vi "Main.vi"(8 "error":errorcluster) -> (0 "Error out":errorcluster)   [LabVIEW 2018, in "S6.lvclass"]
doc: "Use this template to build a simple state machine design pattern. Each state executes code and determines which state to transition to."
uses:
  S6.lvclass
  S6.lvclass/S6.ctl
  Controller/Public Controls/GlobalConfig.ctl
  Controller/Public Controls/S2Config.ctl
  Public Controls/Outputs.ctl
  Controller/Public Controls/TestInfo.ctl
  Public Controls/ReportHeader.ctl
  62a9a080-f0ee-42f1-9851-61b6bd85b26e.vi
  18d9e863-2333-4af4-97b0-9e95cfa094dc.vi
  <vilib>/Utility/file.llb/Write Delimited Spreadsheet (string).vi
  Controller/GUI.lvclass
  IO/IO.lvclass
panel:
  out "Loop":i32
  # "S6 MAIN"
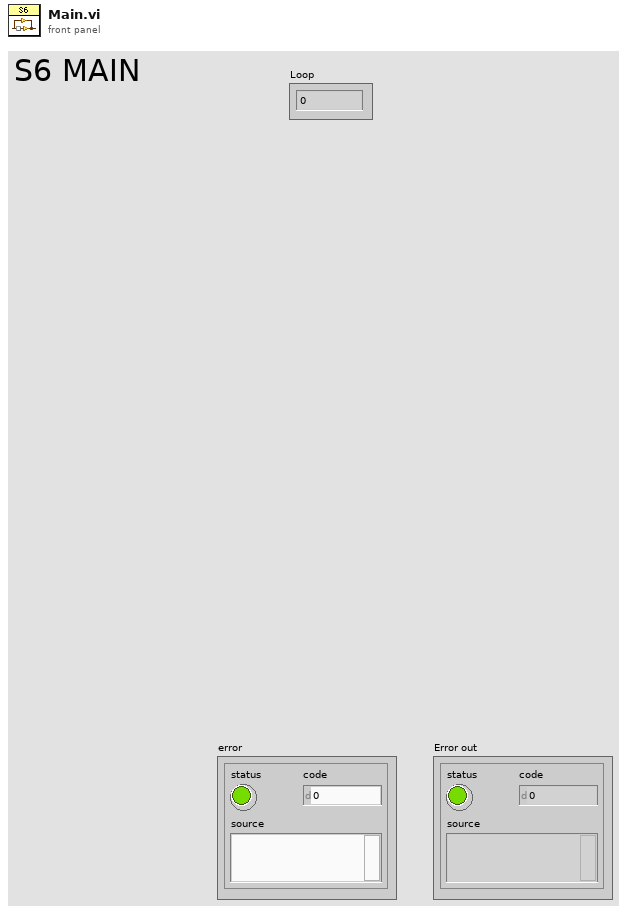
[diagram p1: front panel]
types:
  T1 = typedef "S6.lvclass/Outputs.ctl" = cluster{"LO P":bool, "HI P":bool, "Z3Vent":bool, "V2 Vent":bool, "IsLidLocked":bool}
  T2 = typedef "GUI.lvclass/TestInfo.ctl" = cluster{"TestType":string, "SN":string}
  T3 = typedef "S6.lvclass/ReportHeader.ctl" = string
  T4 = typedef "S6.lvclass/State.ctl" = enum16{"Initialize", "SetConfig", "AckAlarm", "Alarm", "Idle", "LockLid", "LowPressure", "Pressurize", "DecayTest", "Vent", "Abort", "Start", "CreateReports", "WriteToReport", "WritePressure", "Error", "Exit"}
  T5 = typedef "GUI.lvclass/S2Config.ctl" = cluster{"ECLOP_TIMER":dbl, "EC_PTEST_TIMER":dbl, "EC_PSTABLE_WAIT":dbl, "ECZ3_POFF_STABLE":dbl, "EC_PTEST_SCALE_FACTOR":dbl, "EC_PTEST_DELTA_BASELINE":dbl}
  T6 = typedef "GUI.lvclass/GlobalConfig.ctl" = cluster{"Report Folder Path":path, "PT1_MIN":dbl, "PT1_MAX":dbl, "VENT_PMAX":dbl, "LOP_TARGET":dbl, "LOP_RAMP":dbl, "LOP_LEAK_MAX":dbl, "HIP_TARGET":dbl, "HIP_RAMP":dbl, "HIP_MIN":dbl, "HIP_MAX":dbl, "BLEED_TIME":dbl, "LOP_MAX":dbl, "LOP_MIN":dbl, "PT131Com":refnum<visa-resource-name>, "PT231Com":refnum<visa-resource-name>, "PT331Com":refnum<visa-resource-name>, "PT431Com":refnum<visa-resource-name>, "PT531Com":refnum<visa-resource-name>, "PT631Com":refnum<visa-resource-name>}
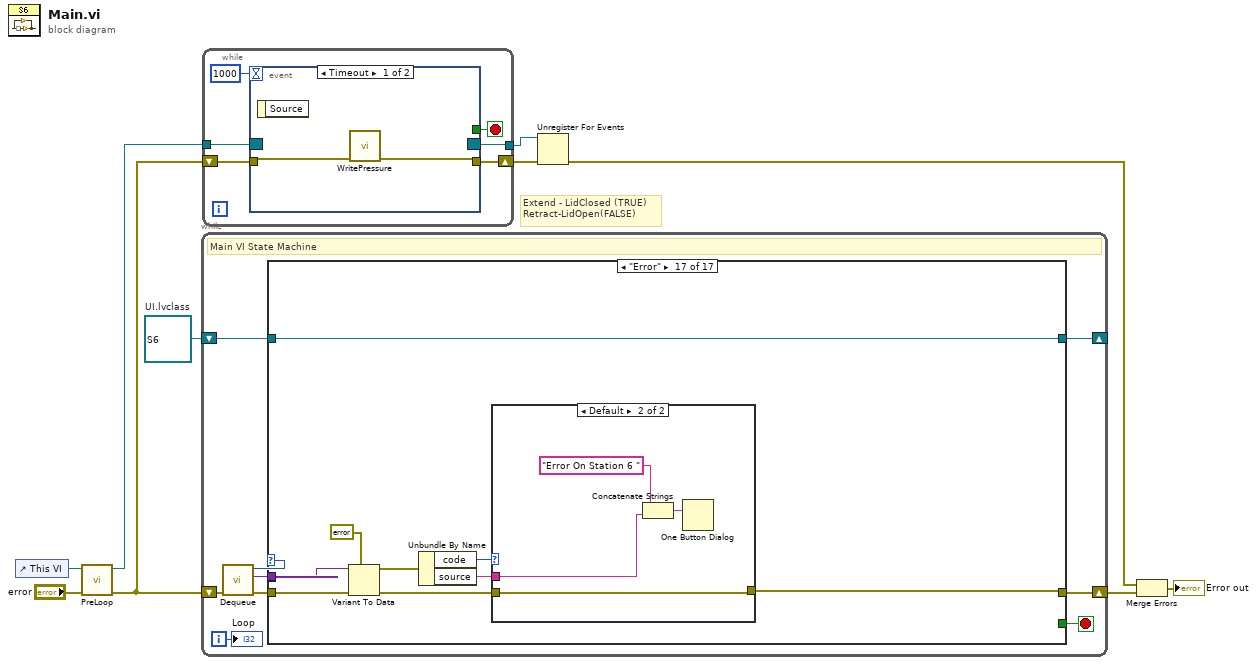
[diagram p0: block diagram]
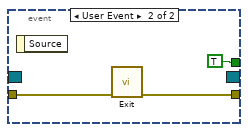
[diagram p2: hidden frame]
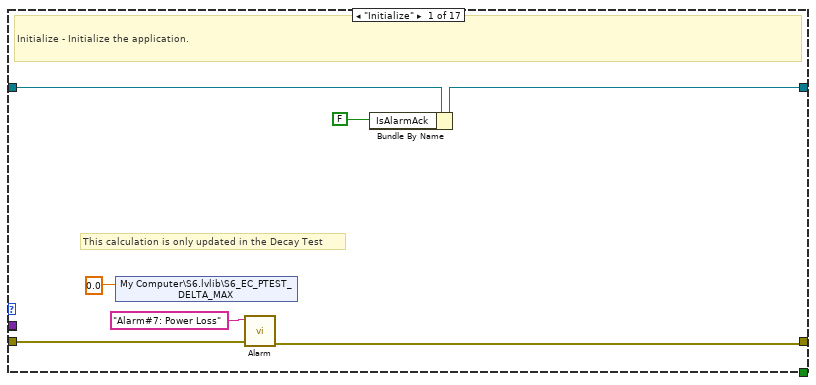
[diagram p3: hidden frame]
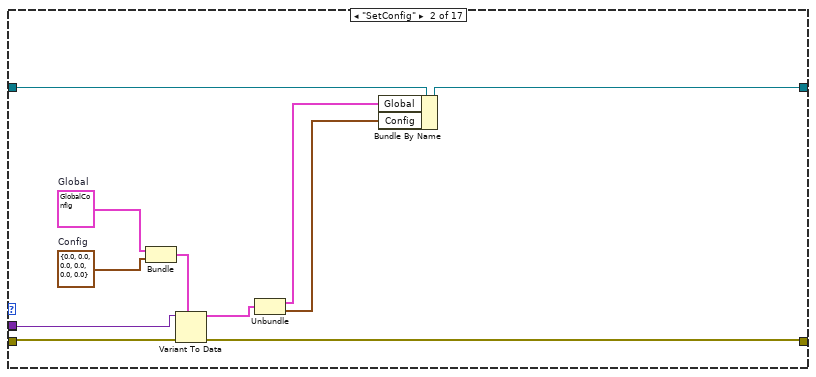
[diagram p4: hidden frame]
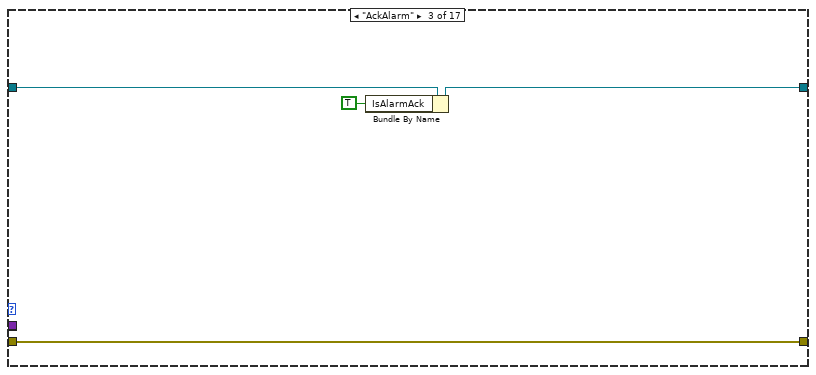
[diagram p5: hidden frame]
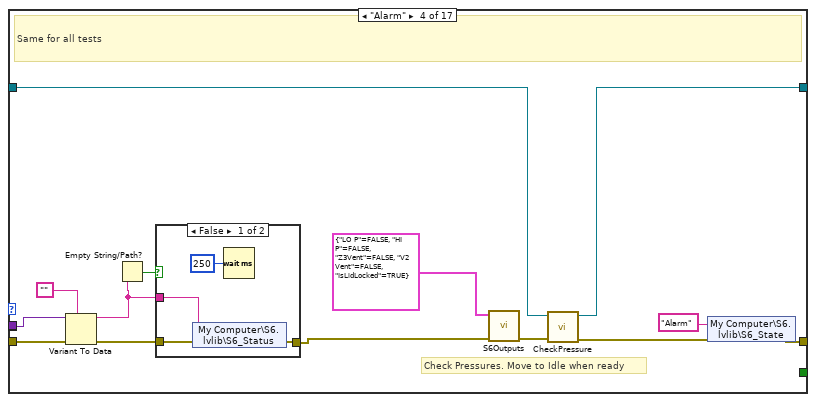
[diagram p6: hidden frame]
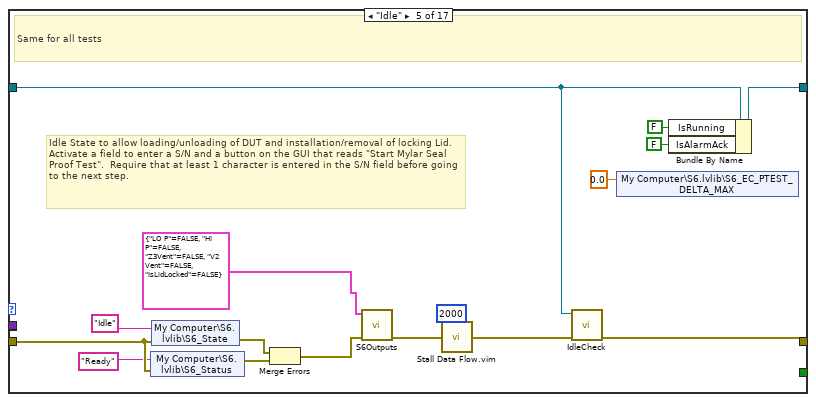
[diagram p8: hidden frame]
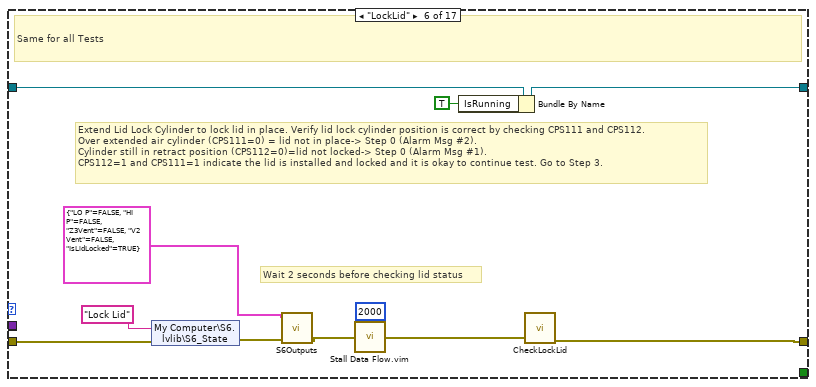
[diagram p9: hidden frame]
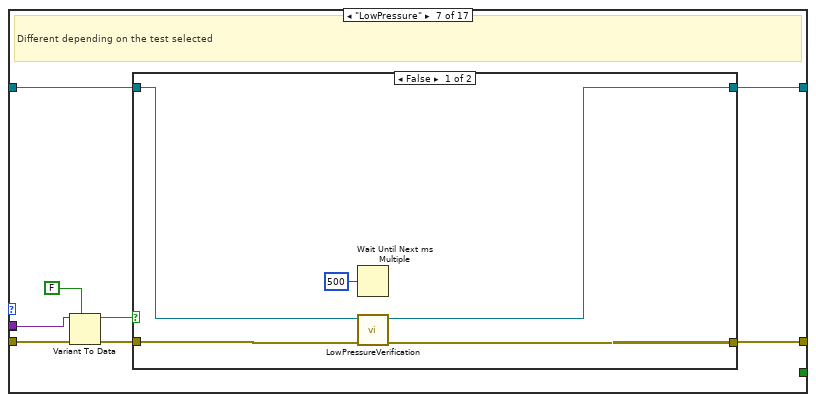
[diagram p10: hidden frame]
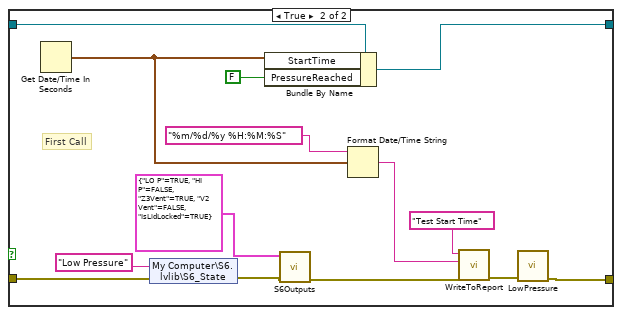
[diagram p11: hidden frame]
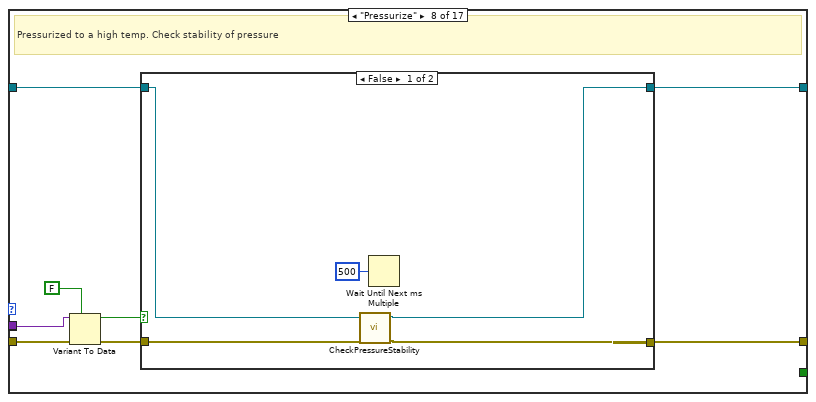
[diagram p12: hidden frame]
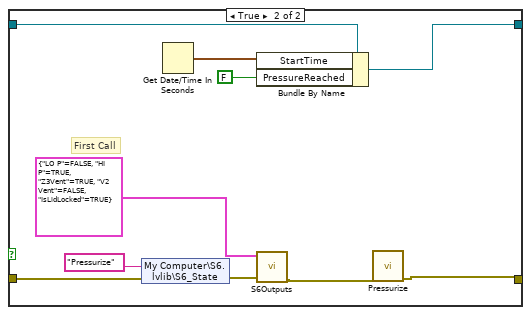
[diagram p13: hidden frame]
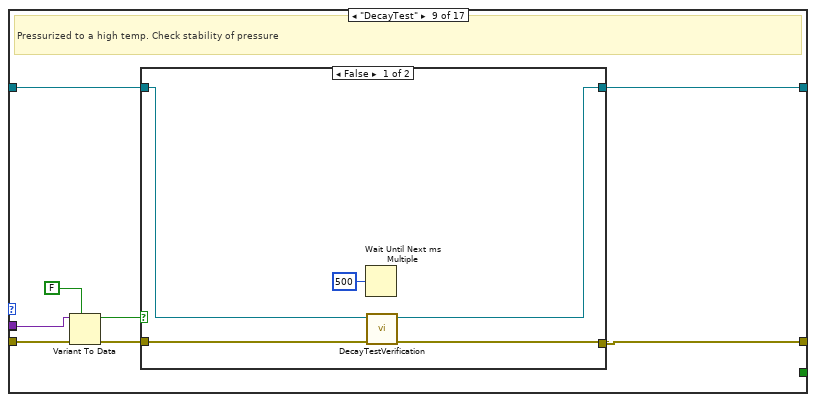
[diagram p14: hidden frame]
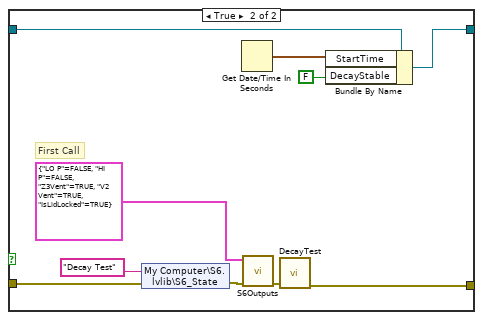
[diagram p15: hidden frame]
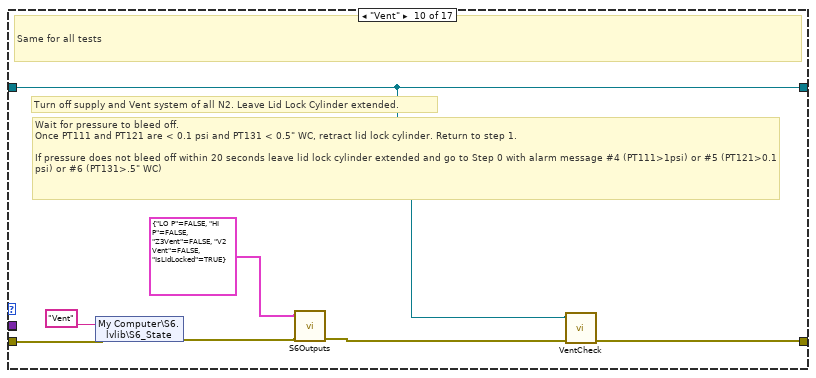
[diagram p16: hidden frame]
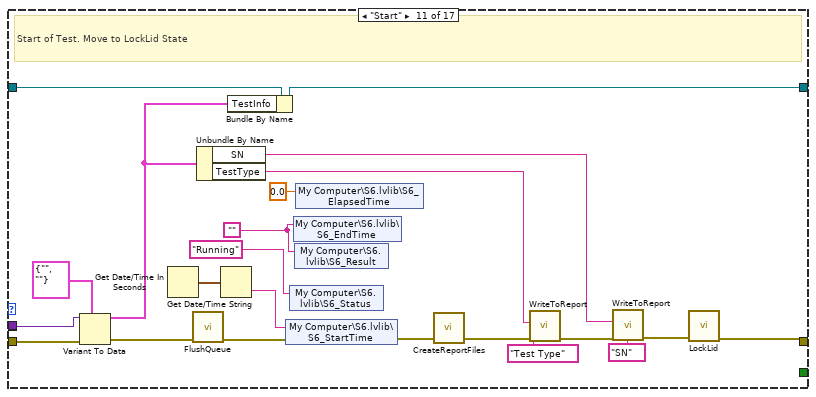
[diagram p17: hidden frame]
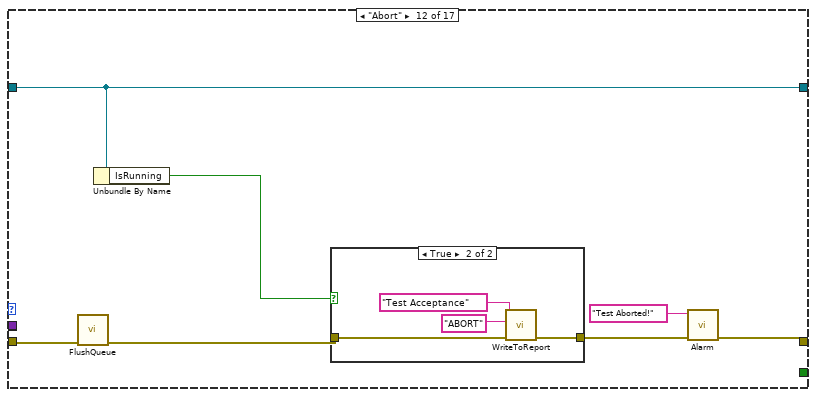
[diagram p18: hidden frame]
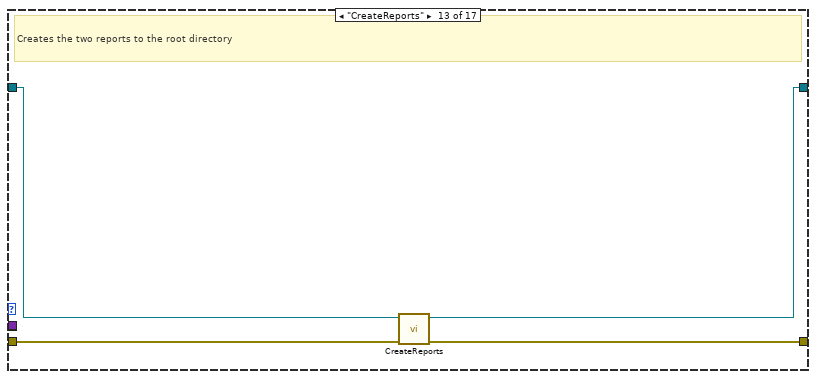
[diagram p20: hidden frame]
diagram:
  w10 = refnum<class "S6.lvclass"> refnum  # UI.lvclass
  # "Extend - LidClosed (TRUE)\nRetract-LidOpen(FALSE)"
  n1 = control-ref of="This VI"() -> (w7:refnum<vi>)
  n2 = call "PreLoop.vi"("error in"="error", "VI Ref"=w7) -> ("error out"=w6:errorcluster, "Event Registration Refnum"=w8:refnum<event-registration>)  [unwired: 8 in]
  n3 = while {
    shift-right: [w19] -> w3
    shift-left: w6 -> [w15]
    shift-right: [w16] -> _
    shift-left: w10 -> [w17]
    i -> [w11]
    stop <- w18 stop-if-true
    # "Main VI State Machine"
    n4 = call "Dequeue.vi"("error in"=w15) -> ("error out"=w14:errorcluster, "Data"=w12:variant, "State"=w13:T4)  [unwired: 8 in]
    n5 = case shown="\"Error\"" w13 {
      tunnel: [_ _ _ _ _ _ _ _ _ _ _ _ _ _ _ w244 _] -> w18
      tunnel: w14 -> [w24 w36 w41 w50 w75 w86 w94 w121 w144 w167 w185 w190 w204 w218 w223 w242 w250]
      tunnel: [w23 w27 w41 w51 w69 w84 w95 w122 w145 w165 w174 w195 w203 w211 w222 w242 w246] -> w19
      tunnel: w17 -> [w26 w37 w40 w54 w65 w87 w89 w116 w139 w164 w189 w194 w205 w217 w225 w243 w253]
      tunnel: [w25 w31 w39 w53 w71 w81 w88 w115 w138 w164 w182 w194 w202 w217 w225 w243 w253] -> w16
      tunnel: w12 -> [_ w32 _ w49 _ _ w93 w120 w143 _ w183 _ _ w219 _ _ w249]
      tunnel: w12 -> [_ _ _ _ _ _ _ _ _ _ _ _ _ _ _ _ _]
      frame "Initialize" {
        # "This calculation is only updated in the Decay Test"
        # "Initialize - Initialize the application."
        n6 = shared-variable "My Computer\\S6.lvlib\\S6_EC_PTEST_DELTA_MAX"(0.0 ("EC_PTEST_DELTA_MAX")) -> ()  [unwired: 1 in, 1 out]
        n7 = call "Alarm.vi"("error in"=w24, "Alarm"="Alarm#7: Power Loss" ("Status")) -> ("error out"=w23:errorcluster)  [unwired: 9 in]
        n8 = Bundle By Name(cluster=w26, "IsAlarmAck"=FALSE) -> (w25:refnum<class "S6.lvclass">)
      }
      frame "SetConfig" {
        w34 = T5 {"ECLOP_TIMER"=0.0, "EC_PTEST_TIMER"=0.0, "EC_PSTABLE_WAIT"=0.0, "ECZ3_POFF_STABLE"=0.0, "EC_PTEST_SCALE_FACTOR"=0.0, "EC_PTEST_DELTA_BASELINE"=0.0}  # Config
        w35 = T6 {"Report Folder Path"=path "", "PT1_MIN"=0.0, "PT1_MAX"=0.0, "VENT_PMAX"=0.0, "LOP_TARGET"=0.0, "LOP_RAMP"=0.0, "LOP_LEAK_MAX"=0.0, "HIP_TARGET"=0.0, "HIP_RAMP"=0.0, "HIP_MIN"=0.0, "HIP_MAX"=0.0, "BLEED_TIME"=0.0, "LOP_MAX"=0.0, "LOP_MIN"=0.0, "PT131Com"="COM5", "PT231Com"="COM6", "PT331Com"="COM7", "PT431Com"="COM8", "PT531Com"="COM9", "PT631Com"="COM10"}  # Global
        n9 = Bundle("Global"=w35, "Config"=w34) -> (w33:cluster{"Global":T6, "Config":T5})  [unwired: 1 in]
        n10 = Variant To Data(error in=w36, type=w33, Variant=w32) -> (data=w30:cluster{"Global":T6, "Config":T5}, error out=w27:errorcluster)
        n11 = Unbundle(w30) -> ("Global"=w29:T6, "Config"=w28:T5)
        n12 = Bundle By Name(cluster=w37, "Global"=w29, "Config"=w28) -> (w31:refnum<class "S6.lvclass">)
      }
      frame "AckAlarm" {
        n13 = Bundle By Name(cluster=w40, "IsAlarmAck"=TRUE) -> (w39:refnum<class "S6.lvclass">)
      }
      frame "Alarm" {
        # "Check Pressures. Move to Idle when ready"
        # "Same for all tests"
        n14 = Variant To Data(error in=w50, type="", Variant=w49) -> (data=w46:string, error out=w45:errorcluster)
        n15 = Empty String/Path?(string/path=w46) -> (empty?=w47:bool)
        n16 = case shown="False" w47 {
          tunnel: w46 -> [w59 _]
          tunnel: w45 -> [w58 w60]
          tunnel: [w57 w60] -> w43
          frame False {
            n17 = shared-variable "My Computer\\S6.lvlib\\S6_Status"(w59, error in=w58) -> (error out=w57:errorcluster)
            n18 = Wait (ms)(milliseconds to wait=u32 250) -> ()  [unwired: 1 out]
          }
          frame True {
          }
        }
        n19 = call "S6Outputs.vi"("error in"=w43, "Outputs"=T1 {"LO P"=FALSE, "HI P"=FALSE, "Z3Vent"=FALSE, "V2 Vent"=FALSE, "IsLidLocked"=TRUE} ("SIOutputs")) -> ("error out"=w42:errorcluster)  [unwired: 9 in]
        n20 = call "CheckPressure.vi"("error in (no error)"=w42, "UI.lvclass"=w54) -> ("error out"=w52:errorcluster, "UI.lvclass 2"=w53:refnum<class "S6.lvclass">)  [unwired: 8 in]
        n21 = shared-variable "My Computer\\S6.lvlib\\S6_State"("Alarm" ("S1Status"), error in=w52) -> (error out=w51:errorcluster)
      }
      frame "Idle" {
        # "Idle State to allow loading/unloading of DUT and installation/removal of locking Lid.  Activate a field to enter a S/N and a button on the GUI that reads \"Start Mylar Seal Proof Test\".  Require that at least 1 character is entered in the S/N field before going to the next step."
        # "Same for all tests"
        n22 = shared-variable "My Computer\\S6.lvlib\\S6_Status"("Ready" ("Status"), error in=w75) -> (error out=w73:errorcluster)
        n23 = shared-variable "My Computer\\S6.lvlib\\S6_State"("Idle" ("S1Status"), error in=w75) -> (error out=w74:errorcluster)
        n24 = Merge Errors(w74, w73) -> (w62:errorcluster)
        n25 = call "S6Outputs.vi"("error in"=w62, "Outputs"=T1 {"LO P"=FALSE, "HI P"=FALSE, "Z3Vent"=FALSE, "V2 Vent"=FALSE, "IsLidLocked"=FALSE} ("SIOutputs")) -> ("error out"=w61:errorcluster)  [unwired: 9 in]
        n26 = call "Stall Data Flow.vim"("value in"=w61, "milliseconds to wait"=u32 2000) -> ("value out"=w67:errorcluster)  [unwired: 1 out]
        n27 = call "IdleCheck.vi"("error in (no error)"=w67, "S2.lvclass"=w65) -> ("error out"=w69:errorcluster)  [unwired: 9 in]
        n28 = shared-variable "My Computer\\S6.lvlib\\S6_EC_PTEST_DELTA_MAX"(0.0 ("EC_PTEST_DELTA_MAX")) -> ()  [unwired: 1 in, 1 out]
        n29 = Bundle By Name(cluster=w65, "IsRunning"=FALSE, "IsAlarmAck"=FALSE) -> (w71:refnum<class "S6.lvclass">)
      }
      frame "LockLid" {
        # "Wait 2 seconds before checking lid status"
        # "Extend Lid Lock Cylinder to lock lid in place. Verify lid lock cylinder position is correct by checking CPS111 and CPS112. \nOver extended air cylinder (CPS111=0) = lid not in place-> Step 0 (Alarm Msg #2). \nCylinder still in retract position (CPS112=0)=lid not locked-> Step 0 (Alarm Msg #1). \nCPS112=1 and CPS111=1 indicate the lid is installed and locked and it is okay to continue test. Go to Step 3."
        # "Same for all Tests"
        n30 = shared-variable "My Computer\\S6.lvlib\\S6_State"("Lock Lid" ("S1Status"), error in=w86) -> (error out=w78:errorcluster)
        n31 = call "S6Outputs.vi"("error in"=w78, "Outputs"=T1 {"LO P"=FALSE, "HI P"=FALSE, "Z3Vent"=FALSE, "V2 Vent"=FALSE, "IsLidLocked"=TRUE} ("SIOutputs")) -> ("error out"=w77:errorcluster)  [unwired: 9 in]
        n32 = call "Stall Data Flow.vim"("value in"=w77, "milliseconds to wait"=u32 2000) -> ("value out"=w83:errorcluster)  [unwired: 1 out]
        n33 = Bundle By Name(cluster=w87, "IsRunning"=TRUE) -> (w81:refnum<class "S6.lvclass">)
        n34 = call "CheckLockLid.vi"("error in (no error)"=w83) -> ("error out"=w84:errorcluster)  [unwired: 10 in]
      }
      frame "LowPressure" {
        # "Different depending on the test selected"
        n35 = Variant To Data(error in=w94, type=FALSE, Variant=w93) -> (data=w90:bool, error out=w91:errorcluster)
        n36 = case shown="False" w90 {
          tunnel: [w99 w104] -> w95
          tunnel: w91 -> [w100 w113]
          tunnel: w89 -> [w98 w110]
          tunnel: [w97 w112] -> w88
          frame False {
            n37 = Wait Until Next ms Multiple(millisecond multiple=u32 500) -> ()  [unwired: 1 out]
            n38 = call "LowPressureVerification.vi"("error in"=w100, "S1 in"=w98) -> ("error out"=w99:errorcluster, "S1 out"=w97:refnum<class "S6.lvclass">)  [unwired: 8 in]
          }
          frame True {
            # "First Call"
            n39 = Get Date/Time In Seconds() -> (seconds since 1Jan1904=w107:timestamp)
            n40 = shared-variable "My Computer\\S6.lvlib\\S6_State"("Low Pressure" ("S1Status"), error in=w113) -> (error out=w102:errorcluster)
            n41 = Bundle By Name(cluster=w110, "StartTime"=w107, "PressureReached"=FALSE ("PT111ReachedPressure")) -> (w112:refnum<class "S6.lvclass">)
            n42 = call "S6Outputs.vi"("error in"=w102, "Outputs"=T1 {"LO P"=TRUE, "HI P"=FALSE, "Z3Vent"=TRUE, "V2 Vent"=FALSE, "IsLidLocked"=TRUE} ("SIOutputs")) -> ("error out"=w101:errorcluster)  [unwired: 9 in]
            n43 = Format Date/Time String(time format string (%c)="%m/%d/%y %H:%M:%S", seconds (now)=w107) -> (date/time string=w106:string)  [unwired: 1 in]
            n44 = call "WriteToReport.vi"("error in"=w101, "Value"=w106, "Header"="Test Start Time" ("S1Status")) -> ("error out"=w105:errorcluster)  [unwired: 8 in]
            n45 = call "LowPressure.vi"("error in"=w105) -> ("error out"=w104:errorcluster)  [unwired: 10 in]
          }
        }
      }
      frame "Pressurize" {
        # "Pressurized to a high temp. Check stability of pressure"
        n46 = Variant To Data(error in=w121, type=FALSE, Variant=w120) -> (data=w117:bool, error out=w118:errorcluster)
        n47 = case shown="False" w117 {
          tunnel: [w124 w131] -> w122
          tunnel: w118 -> [w125 w136]
          tunnel: w116 -> [w127 w132]
          tunnel: [w126 w135] -> w115
          frame False {
            n48 = call "CheckPressureStability.vi"("error in"=w125, "S1 in"=w127) -> ("error out"=w124:errorcluster, "S1 out"=w126:refnum<class "S6.lvclass">)  [unwired: 8 in]
            n49 = Wait Until Next ms Multiple(millisecond multiple=u32 500) -> ()  [unwired: 1 out]
          }
          frame True {
            # "First Call"
            n50 = shared-variable "My Computer\\S6.lvlib\\S6_State"("Pressurize" ("S1Status"), error in=w136) -> (error out=w129:errorcluster)
            n51 = Get Date/Time In Seconds() -> (seconds since 1Jan1904=w134:timestamp)
            n52 = Bundle By Name(cluster=w132, "StartTime"=w134, "PressureReached"=FALSE ("PT111ReachedPressure")) -> (w135:refnum<class "S6.lvclass">)
            n53 = call "S6Outputs.vi"("error in"=w129, "Outputs"=T1 {"LO P"=FALSE, "HI P"=TRUE, "Z3Vent"=TRUE, "V2 Vent"=FALSE, "IsLidLocked"=TRUE} ("SIOutputs")) -> ("error out"=w128:errorcluster)  [unwired: 9 in]
            n54 = call "Pressurize.vi"("error in"=w128) -> ("error out"=w131:errorcluster)  [unwired: 10 in]
          }
        }
      }
      frame "DecayTest" {
        # "Pressurized to a high temp. Check stability of pressure"
        n55 = Variant To Data(error in=w144, type=FALSE, Variant=w143) -> (data=w140:bool, error out=w141:errorcluster)
        n56 = case shown="False" w140 {
          tunnel: [w147 w155] -> w145
          tunnel: w141 -> [w148 w159]
          tunnel: w139 -> [w150 w156]
          tunnel: [w149 w158] -> w138
          frame False {
            n57 = Wait Until Next ms Multiple(millisecond multiple=u32 500) -> ()  [unwired: 1 out]
            n58 = call "DecayTestVerification.vi"("error in"=w148, "ClassDataIn"=w150) -> ("error out"=w147:errorcluster, "S1 out"=w149:refnum<class "S6.lvclass">)  [unwired: 8 in]
          }
          frame True {
            # "First Call"
            n59 = shared-variable "My Computer\\S6.lvlib\\S6_State"("Decay Test" ("S1Status"), error in=w159) -> (error out=w152:errorcluster)
            n60 = Get Date/Time In Seconds() -> (seconds since 1Jan1904=w157:timestamp)
            n61 = call "S6Outputs.vi"("error in"=w152, "Outputs"=T1 {"LO P"=FALSE, "HI P"=FALSE, "Z3Vent"=TRUE, "V2 Vent"=TRUE, "IsLidLocked"=TRUE} ("SIOutputs")) -> ("error out"=w151:errorcluster)  [unwired: 9 in]
            n62 = call "DecayTest.vi"("error in"=w151) -> ("error out"=w155:errorcluster)  [unwired: 10 in]
            n63 = Bundle By Name(cluster=w156, "StartTime"=w157, "DecayStable"=FALSE) -> (w158:refnum<class "S6.lvclass">)
          }
        }
      }
      frame "Vent" {
        # "Wait for pressure to bleed off. \nOnce PT111 and PT121 are < 0.1 psi and PT131 < 0.5\" WC, retract lid lock cylinder. Return to step 1. \n\nIf pressure does not bleed off within 20 seconds leave lid lock cylinder extended and go to Step 0 with alarm message #4 (PT111>1psi) or #5 (PT121>0.1 psi) or #6 (PT131>.5\" WC)"
        # "Turn off supply and Vent system of all N2. Leave Lid Lock Cylinder extended."
        # "Same for all tests"
        n64 = shared-variable "My Computer\\S6.lvlib\\S6_State"("Vent" ("S1Status"), error in=w167) -> (error out=w162:errorcluster)
        n65 = call "S6Outputs.vi"("error in"=w162, "Outputs"=T1 {"LO P"=FALSE, "HI P"=FALSE, "Z3Vent"=FALSE, "V2 Vent"=FALSE, "IsLidLocked"=TRUE} ("SIOutputs")) -> ("error out"=w161:errorcluster)  [unwired: 9 in]
        n66 = call "VentCheck.vi"("error in (no error)"=w161, "S2.lvclass"=w164) -> ("error out"=w165:errorcluster)  [unwired: 9 in]
      }
      frame "Start" {
        w171 = ""
        # "Start of Test. Move to LockLid State"
        n67 = Variant To Data(error in=w185, type=T2 {"TestType"="", "SN"=""} ("TestInfo"), Variant=w183) -> (data=w179:T2, error out=w169:errorcluster)
        n68 = Get Date/Time In Seconds() -> (seconds since 1Jan1904=w188:timestamp)
        n69 = call "FlushQueue.vi"("error in"=w169) -> ("error out"=w168:errorcluster)  [unwired: 10 in]
        n70 = Unbundle By Name(w179) -> ("SN"=w177:string, "TestType"=w170:string)
        n71 = Get Date/Time String(seconds (now)=w188) -> (time string=w187:string)  [unwired: 2 in, 1 out]
        n72 = Bundle By Name(cluster=w189, "TestInfo"=w179) -> (w182:refnum<class "S6.lvclass">)
        n73 = shared-variable "My Computer\\S6.lvlib\\S6_StartTime"(w187, error in=w168) -> (error out=w173:errorcluster)
        n74 = shared-variable "My Computer\\S6.lvlib\\S6_Status"("Running" ("S1Status")) -> ()  [unwired: 1 in, 1 out]
        n75 = shared-variable "My Computer\\S6.lvlib\\S6_EndTime"(w171) -> ()  [unwired: 1 in, 1 out]
        n76 = shared-variable "My Computer\\S6.lvlib\\S6_Result"(w171) -> ()  [unwired: 1 in, 1 out]
        n77 = shared-variable "My Computer\\S6.lvlib\\S6_ElapsedTime"(0.0 ("ElapsedTime")) -> ()  [unwired: 1 in, 1 out]
        n78 = call "CreateReportFiles.vi"("error in"=w173) -> ("error out"=w180:errorcluster)  [unwired: 10 in]
        n79 = call "WriteToReport.vi"("error in"=w180, "Value"=w170, "Header"="Test Type") -> ("error out"=w178:errorcluster)  [unwired: 8 in]
        n80 = call "WriteToReport.vi"("error in"=w178, "Value"=w177, "Header"="SN") -> ("error out"=w175:errorcluster)  [unwired: 8 in]
        n81 = call "LockLid.vi"("error in"=w175) -> ("error out"=w174:errorcluster)  [unwired: 10 in]
      }
      frame "Abort" {
        n82 = call "FlushQueue.vi"("error in"=w190) -> ("error out"=w192:errorcluster)  [unwired: 10 in]
        n83 = Unbundle By Name(w194) -> ("IsRunning"=w193:bool)
        n84 = case shown="True" w193 {
          tunnel: w192 -> [w197 w201]
          tunnel: [w197 w200] -> w196
          frame False {
          }
          frame True {
            n85 = call "WriteToReport.vi"("error in"=w201, "Value"="ABORT", "Header"=T3 "Test Acceptance") -> ("error out"=w200:errorcluster)  [unwired: 8 in]
          }
        }
        n86 = call "Alarm.vi"("error in"=w196, "Alarm"="Test Aborted!" ("S1Status")) -> ("error out"=w195:errorcluster)  [unwired: 9 in]
      }
      frame "CreateReports" {
        # "Creates the two reports to the root directory"
        n87 = call "CreateReports.vi"("error in (no error)"=w204, "S1 in"=w205) -> ("error out"=w203:errorcluster, "S1 out"=w202:refnum<class "S6.lvclass">)  [unwired: 8 in]
      }
      frame "WriteToReport" {
        n88 = Variant To Data(error in=w218, type="", Variant=w219) -> (data=w214:string, error out=w215:errorcluster)
        n89 = Unbundle By Name(w217) -> ("TestReport"=w216:path)
        n90 = Open/Create/Replace File(file path (use dialog)=w216, error in=w215) -> (refnum out=w207:refnum<file>, error out=w210:errorcluster)  [unwired: 4 in, 1 out]
        n91 = Set File Position(refnum=w207, from (0:start)=enum16{"start", "end", "current"}."end", error in=w210) -> (refnum out=w206:refnum<file>, error out=w208:errorcluster)  [unwired: 1 in]
        n92 = Write to Text File(file (use dialog)=w206, text=w214, error in=w208) -> (refnum out=w213:refnum<file>, error out=w212:errorcluster)  [unwired: 1 in, 1 out]
        n93 = Close File(refnum=w213, error in=w212) -> (error out=w211:errorcluster)  [unwired: 1 out]
      }
      frame "WritePressure" {
        n94 = Unbundle By Name(w225) -> ("PressureReport"=w224:path, "IsRunning"=w221:bool)
        n95 = case shown="True" w221 {
          tunnel: w224 -> [_ w233]
          tunnel: w223 -> [w226 w232]
          tunnel: [w226 w231] -> w222
          frame False {
          }
          frame True {
            n96 = shared-variable "My Computer\\S6.lvlib\\S6_EC_PTEST_DELTA_MAX"() -> (w228:dbl)  [unwired: 1 in, 1 out]
            n97 = shared-variable "My Computer\\S6.lvlib\\S6_PT631"() -> (w238:dbl)  [unwired: 1 in, 1 out]
            n98 = shared-variable "My Computer\\S6.lvlib\\S6_PT621"() -> (w239:dbl)  [unwired: 1 in, 1 out]
            n99 = Get Date/Time In Seconds() -> (seconds since 1Jan1904=w241:timestamp)
            n100 = Number To Fractional String(number=w228) -> (F-format string=w227:string)  [unwired: 3 in]
            n101 = Number To Fractional String(number=w239) -> (F-format string=w236:string)  [unwired: 3 in]
            n102 = Number To Fractional String(number=w238) -> (F-format string=w235:string)  [unwired: 3 in]
            n103 = Format Date/Time String(time format string (%c)="%m/%d/%y %H:%M:%S", seconds (now)=w241) -> (date/time string=w237:string)  [unwired: 1 in]
            n104 = Build Array(w237, w236, w235, w227) -> (w234:string[])
            n105 = call-poly <vilib>:"Write Delimited Spreadsheet.vi"("file path (dialog if empty)"=w233, "1D data"=w234, "append to file? (new file:F)"=TRUE, "error in (no error)"=w232, "delimiter (\\t)"="," ("delimiter (\\t)")) -> ("error out"=w231:errorcluster)  [unwired: 9 in, 1 out]
          }
        }
      }
      frame "Exit" {
        w244 = TRUE  # Stop Loop
        # "Exit - Exit the application.\nSave / Close any files"
      }
      frame "Error" {
        n106 = Variant To Data(error in=w250, type=errorcluster {"status"=FALSE, "code"=0, "source"=""} ("error out"), Variant=w249) -> (data=w251:errorcluster, error out=w247:errorcluster)
        n107 = Unbundle By Name(w251) -> ("code"=w245:i32, "source"=w248:string)
        n108 = case shown="Default" w245 {
          tunnel: w248 -> [_ w255]
          tunnel: w247 -> [w254 w258]
          tunnel: [w254 w258] -> w246
          frame 1 {
            # "Error talking to other modules. \n\nIgnore. If testing by itself."
          }
          frame Default {
            n109 = Concatenate Strings("Error On Station 6 ", w255) -> (w257:string)
            n110 = One Button Dialog(message=w257) -> ()  [unwired: 1 in, 1 out]
          }
        }
      }
    }
    "Loop" <- w11
  }
  n111 = while {
    tunnel: w8 -> [w260]
    shift-right: [w262] -> w5
    shift-left: w6 -> [w264]
    tunnel: [w261] -> w4
    stop <- w263 stop-if-true
    n112 = event shown="[0] Timeout" {
      selector: w260 -> [_ _]
      dyn-events: [_ _] -> w261
      timeout: 1000 -> [_ _]
      tunnel: w264 -> [w266 w269]
      tunnel: [w265 w268] -> w262
      tunnel: [_ TRUE] -> w263
      event Timeout {
        n113 = event-data() -> ()  [unwired: 1 in, 1 out]
        n114 = call "WritePressure.vi"("error in"=w266) -> ("error out"=w265:errorcluster)  [unwired: 10 in]
      }
      event User Event {
        n115 = event-data() -> ()  [unwired: 1 in, 1 out]
        n116 = call "Exit.vi"("error in"=w269) -> ("error out"=w268:errorcluster)  [unwired: 10 in]
      }
    }
  }
  n117 = Unregister For Events(event registration refnum=w4, error in=w5) -> (error out=w2:errorcluster)
  n118 = Merge Errors(w2, w3) -> (→"Error out":errorcluster)
